vi "Split ChildPanel.vi"(7 "Split Mode":T1, 8 "error in":errorcluster caption="错误输入（无错误）", 10 "L/R Child":i32, 11 "PanelDataNode.lvclass":refnum<class "PanelDataNode.lvclass">) -> (0 "error out":errorcluster, 3 "PanelLinkNode输出":refnum<class "PanelDataNode.lvclass">)   [LabVIEW 2013, in "PanelDataNode.lvclass"]
uses:
  PanelDataNode.lvclass
  Split Mode.ctl
  PanelLinkNode/PanelLinkNode.lvclass/PanelLinkNode.ctl
  PanelLinkNode/PanelLinkNode.lvclass
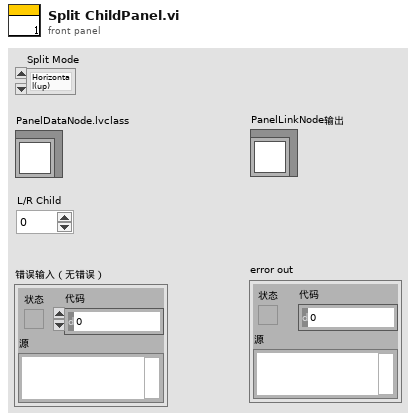
[diagram p1: front panel]
types:
  T1 = typedef "PanelDataNode.lvclass/Split Mode.ctl" = enum16{"Horizontal(up)", "Vertical(left)", "Horizontal(down)", "Vertical(right)"}
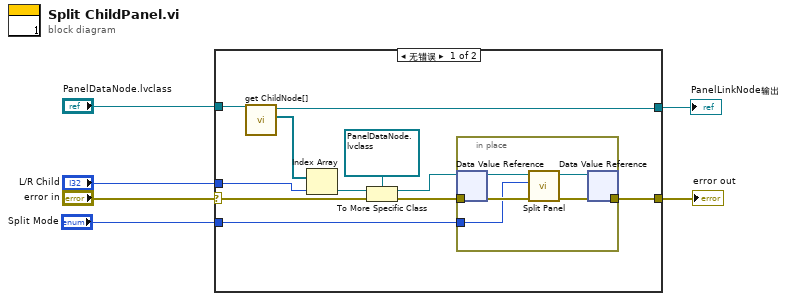
[diagram p0: block diagram]
diagram:
  n1 = case shown="无错误" "error in" {
    selector: "error in" -> [w11 w23]
    tunnel: "PanelDataNode.lvclass" -> [w13 w24]
    tunnel: [w12 w24] -> w5
    tunnel: [w9 w23] -> w3
    tunnel: "L/R Child" -> [w8 _]
    tunnel: "Split Mode" -> [w7 _]
    frame No Error {
      n2 = call "get ChildNode[].vi"("PanelLinkNode输入"=w13) -> ("ChildNode*[]"=w15:refnum<data-value>[], "PanelLinkNode输出"=w12:refnum<class "PanelDataNode.lvclass">)  [unwired: 8 in, 1 out]
      n3 = Index Array(array=w15, index=w8) -> (element=w14:refnum<data-value>)
      n4 = To More Specific Class(target class=refnum<data-value> refnum ("Node*"), reference=w14, error in=w11) -> (specific class reference=w16:refnum<data-value>, error out=w10:errorcluster)
      n5 = in-place {
        in-place-border: w10 -> [w20]
        in-place-border: [w19] -> w9
        in-place-border: w7 -> [w18]
        n6 = in-place-dvr #1(w16) -> (w22:refnum<class "PanelDataNode.lvclass">)  [unwired: 1 out]
        n7 = call-dynamic "Split Panel.vi"("error in (no error)"=w20, "Split Mode"=w18, "PanelDataNode 输入"=w22) -> ("error out"=w19:errorcluster, "PanelDataNode 输出"=w21:refnum<class "PanelDataNode.lvclass">)  [unwired: 6 in, 1 out]
        n8 = in-place-dvr #1(w21) -> ()  [unwired: 2 out]
      }
    }
    frame Error {
    }
  }
  "PanelLinkNode输出" <- w5
  "error out" <- w3
